vi "Publish Events.vi"(8 "error in (no error)":errorcluster, 10 "Events":T1[](array[typedef]), 11 "Event Reporter Module in":refnum<class "Event Reporter Module.lvclass">) -> (0 "error out":errorcluster, 3 "Event Reporter Module out":refnum<class "Event Reporter Module.lvclass">)   [LabVIEW 2020, in "Volatus.lvlib" / "Event Reporter Module.lvclass"]
uses:
  Event Reporter Module.lvclass
  Event.ctl
  Event Level.ctl
  Event Reporter Module.lvclass/Event Reporter Module.ctl
  Module/Module.lvclass/Module.ctl
  VolatusAPI/VolatusAPI.lvclass/VolatusAPI.ctl
  Message Forward (ID).ctl
  Volatus.lvlib
  MessageQ/MessageQ.lvclass
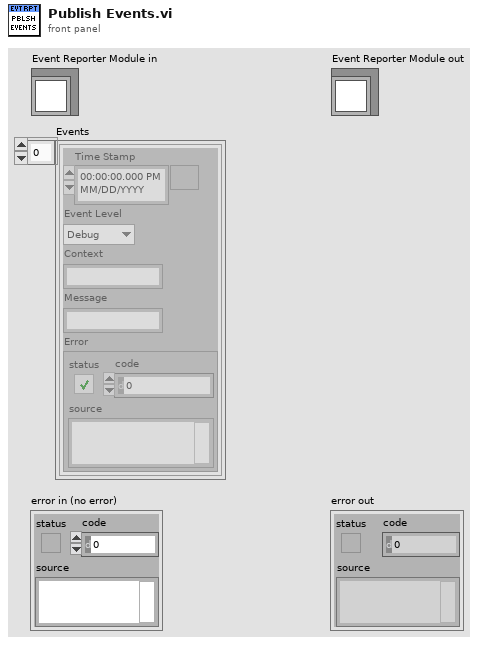
[diagram p1: front panel]
types:
  T1 = typedef "Volatus.lvlib/Event.ctl" = cluster{"Time Stamp":timestamp, "Event Level":T2, "Context":string, "Message":string, "Error":errorcluster}
  T2 = typedef "Volatus.lvlib/Event Level.ctl" = enum16{"Debug", "Info", "Warning", "Error"}
  T3 = typedef "Volatus.lvlib/Message Forward (ID).ctl" = cluster{"Node ID":u32, "Type":string, "Payload":u8[]}
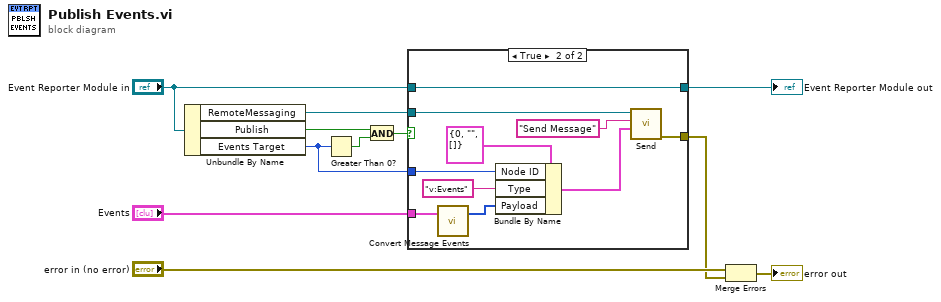
[diagram p0: block diagram]
diagram:
  n1 = Unbundle By Name("Event Reporter Module in") -> ("RemoteMessaging"=w3:refnum<class "MessageQ.lvclass">, "Publish"=w6:bool, "Events Target"=w2:u32)
  n2 = Greater Than 0?(x=w2) -> (x > 0?=w5:bool)
  n3 = And(x=w6, y=w5) -> (x .and. y?=w4:bool)
  n4 = case shown="True" w4 {
    tunnel: "Event Reporter Module in" -> [w12 w21]
    tunnel: [w12 w21] -> w9
    tunnel: "Events" -> [_ w22]
    tunnel: w3 -> [_ w16]
    tunnel: w2 -> [_ w17]
    tunnel: [_ w13] -> w1
    frame False {
      # "No publishing for events"
    }
    frame True {
      n5 = call "Convert Message Events.vi"("Local Events"=w22) -> ("Payload"=w18:u8[])  [unwired: 6 in]
      n6 = Bundle By Name(cluster=T3 {"Node ID"=0, "Type"="", "Payload"=[]} ("Message Forward (ID)"), "Node ID"=w17, "Type"="v:Events", "Payload"=w18) -> (w15:T3)
      n7 = call "Send.vi"("Data"=w15, "ID"="Send Message", "MessageQ in"=w16) -> ("error out"=w13:errorcluster)  [unwired: 7 in, 1 out]
    }
  }
  "Event Reporter Module out" <- w9
  n8 = Merge Errors("error in (no error)", w1) -> (→"error out":errorcluster)
